vi "XY to (x,y) (multiple).vi"(8 "error in (no error)":errorcluster, 11 "XY-data":cluster{"X-array":dbl[], "Y-array":dbl[]}[](array[cluster]) {"Y-array" format="%.2p"; "X-array" format="%.2p"}) -> (0 "error out":errorcluster, 2 "[[(x,y)]]":cluster{"x":dbl, "y":dbl}[][](array[cluster]), 3 "XY-data out":cluster{"X-array":dbl[], "Y-array":dbl[]}[](array[cluster]) {"Y-array" format="%.2p"; "X-array" format="%.2p"})   [LabVIEW 2019, in "xy_utilities.lvlib"]
doc: "Convert <b>XY-data</b> (cluster of arrays of X and Y) to <b>(x,y)</b> coordinates (array of clusters of (x,y) values).\n\nWire data to the data input to determine the polymorphic instance to use or manually select the instance."
uses:
  xy_utilities.lvlib
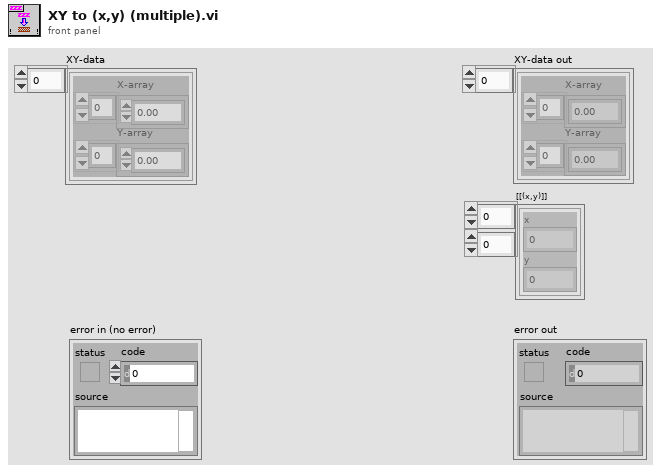
[diagram p1: front panel]
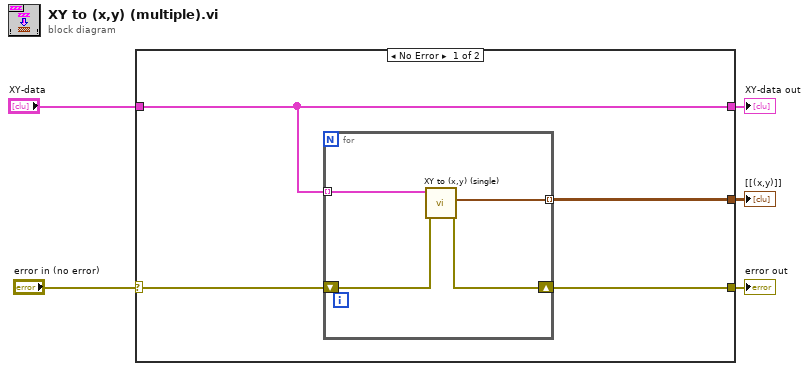
[diagram p0: block diagram]
diagram:
  n1 = case shown="No Error" "error in (no error)" {
    selector: "error in (no error)" -> [w9 w15]
    tunnel: [w8 w15] -> w4
    tunnel: "XY-data" -> [w6 w14]
    tunnel: [w6 w14] -> w2
    tunnel: [w7 _] -> w1
    frame No Error {
      n2 = for {
        shift-right: [w12] -> w8
        shift-left: w9 -> [w13]
        tunnel: w6 -> [w11] mode=indexing
        tunnel: [w10] -> w7 mode=indexing
        n3 = call "XY to (x,y) (single).vi"("error in (no error)"=w13, "XY-data"=w11) -> ("error out"=w12:errorcluster, "[(x,y)]"=w10:cluster{"x":dbl, "y":dbl}[])  [unwired: 7 in, 1 out]
      }
    }
    frame Error {
    }
  }
  "error out" <- w4
  "XY-data out" <- w2
  "[[(x,y)]]" <- w1
